vi "main_entrance.vi"   [LabVIEW 2020]
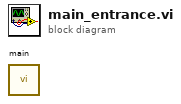
[diagram p0: block diagram]
diagram:
  n1 = call "main.vi"() -> ()  [unwired: 12 in]
